vi "4310 DMM Measure.vi"(0 "IVI Refnum in":refnum<k15>, 1 "task in":refnum<k21>, 2 "Number of Samples in":i32, 3 "error in":errorcluster, 4 "gRPCid":T1) -> (7 "IVI Refnum out":refnum<k15>, 8 "task out":refnum<k21>, 9 "STOPSTREAM?":bool=TRUE, 10 "error out":errorcluster)   [LabVIEW 2019]
uses:
  VIs/grpcId.ctl
  QueryServer_AnalogInputData.ctl
  Global Operations.ctl
  <vilib>/DAQmx/read.llb/DAQmx Read (Analog 1D Wfm NChan NSamp).vi
  <vilib>/DAQmx/miscellaneous.llb/DAQmx Fill In Error Info.vi
  labview-grpc-query-server.lvlib
  <vilib>/NI_Real-Time Target Support.lvlib
  VIs/gprc-support.lvlib
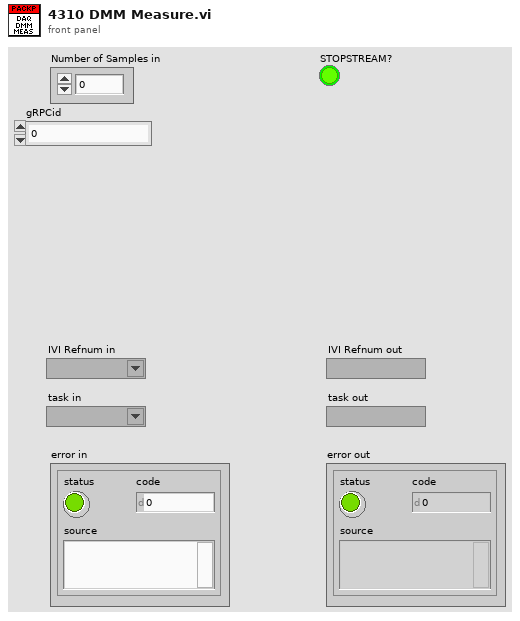
[diagram p1: front panel]
types:
  T1 = typedef "gprc-support.lvlib/grpcId.ctl" = u64
  T2 = typedef "Global Operations.ctl" = enum16{"Get", "Set"}
  T3 = typedef "labview-grpc-query-server.lvlib/QueryServer_AnalogInputData.ctl" = cluster{"RepeatedDMMValue":sgl[], "RepeatedDAQValue0":sgl[], "RepeatedDAQValue1":sgl[], "RepeatedDAQValue2":sgl[], "RepeatedDAQValue3":sgl[], "RepeatedDAQValue4":sgl[], "RepeatedDAQValue5":sgl[], "RepeatedDAQValue6":sgl[], "RepeatedDAQValue7":sgl[], "t0":string, "dt":sgl, "errorstatus":bool, "errorcode":i32, "errorsource":string}
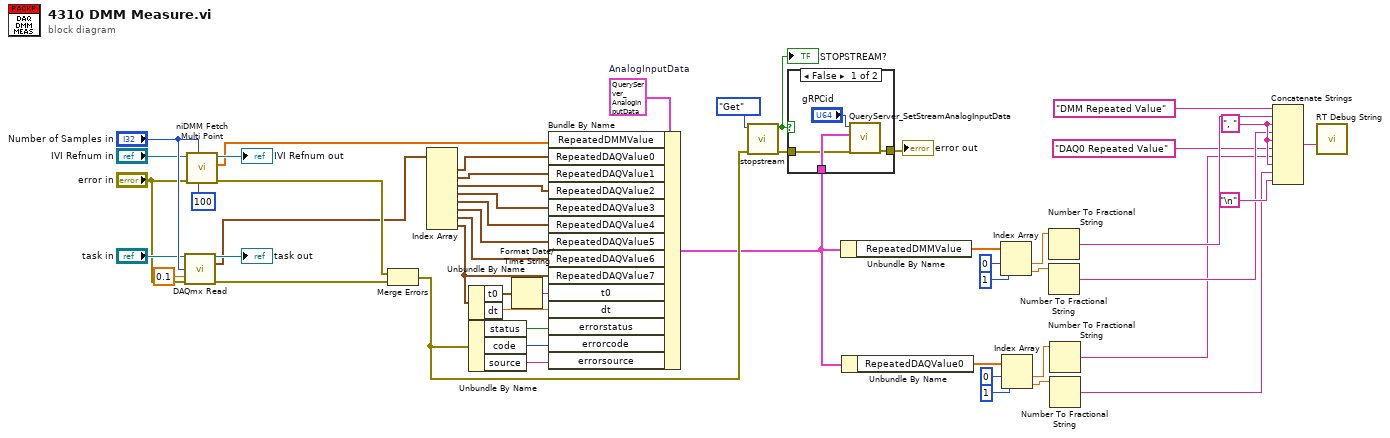
[diagram p0: block diagram]
diagram:
  w13 = ", "
  w43 = T3 {"RepeatedDMMValue"=[], "RepeatedDAQValue0"=[], "RepeatedDAQValue1"=[], "RepeatedDAQValue2"=[], "RepeatedDAQValue3"=[], "RepeatedDAQValue4"=[], "RepeatedDAQValue5"=[], "RepeatedDAQValue6"=[], "RepeatedDAQValue7"=[], "t0"="", "dt"=0.0, "errorstatus"=FALSE, "errorcode"=0, "errorsource"=""}  # AnalogInputData
  n1 = call-poly <vilib>:"DAQmx Read.vi"("task/channels in"="task in", "number of samples per channel"="Number of Samples in", "timeout"=0.1, "error in"="error in") -> ("task out"=→"task out":refnum<k21>, "data"=w29:waveform(dbl)[], "error out"=w45:errorcluster)  [unwired: 9 in]
  n2 = call <instrlib>:"niDMM Fetch Multi Point.vi"("Maximum Time (msec)"=100, "Number to Fetch"="Number of Samples in", "error in (no error)"="error in", "instrument handle"="IVI Refnum in") -> ("error out"=w44:errorcluster, "Measurements"=w30:dbl[], "instrument handle out"=→"IVI Refnum out":refnum<k15>)  [unwired: 4 in, 1 out]
  n3 = Merge Errors(w44, w45) -> (w21:errorcluster)
  n4 = Index Array(array=w29) -> (element #1=w42:waveform(dbl), element #2=w41:waveform(dbl), element #3=w40:waveform(dbl), element #4=w39:waveform(dbl), element #5=w38:waveform(dbl), element #6=w37:waveform(dbl), element #7=w36:waveform(dbl), element #8=w35:waveform(dbl))  [unwired: 8 in]
  n5 = Unbundle By Name(w35) -> ("t0"=w34:timestamp, "dt"=w32:dbl)
  n6 = Unbundle By Name(w21) -> ("status"=w27:bool, "code"=w31:i32, "source"=w26:string)
  n7 = Format Date/Time String(seconds (now)=w34) -> (date/time string=w33:string)  [unwired: 2 in]
  n8 = Bundle By Name(cluster=w43, "RepeatedDMMValue"=w30, "RepeatedDAQValue0"=w42, "RepeatedDAQValue1"=w41, "RepeatedDAQValue2"=w40, "RepeatedDAQValue3"=w39, "RepeatedDAQValue4"=w38, "RepeatedDAQValue5"=w37, "RepeatedDAQValue6"=w36, "RepeatedDAQValue7"=w35, "t0"=w33, "dt"=w32, "errorstatus"=w27, "errorcode"=w31, "errorsource"=w26) -> (w8:T3)
  n9 = call "stopstream.vi"("error in (no error)"=w21, "Operation"=Global_Operations."Get") -> ("error out"=w22:errorcluster, "STOPSTREAM?"=w23:bool)  [unwired: 8 in]
  "STOPSTREAM?" <- w23
  n10 = case shown="False" w23 {
    tunnel: w8 -> [w56 _]
    tunnel: [w54 w57] -> w25
    tunnel: w22 -> [w53 w57]
    frame False {
      n11 = call "QueryServer_SetStreamAnalogInputData.vi"("error in (no error)"=w53, "AnalogInputData"=w56, "gRPCid"="gRPCid") -> ("error out"=w54:errorcluster)  [unwired: 5 in, 1 out]
    }
    frame True {
    }
  }
  "error out" <- w25
  n12 = Unbundle By Name(w8) -> ("RepeatedDMMValue"=w20:sgl[])
  n13 = Unbundle By Name(w8) -> ("RepeatedDAQValue0"=w3:sgl[])
  n14 = Index Array(array=w20, index #1=0 ("index"), index #2=1 ("index")) -> (element #1=w16:sgl, element #2=w17:sgl)
  n15 = Index Array(array=w3, index #1=0 ("index"), index #2=1 ("index")) -> (element #1=w4:sgl, element #2=w5:sgl)
  n16 = Number To Fractional String(number=w16) -> (F-format string=w11:string)  [unwired: 3 in]
  n17 = Number To Fractional String(number=w17) -> (F-format string=w10:string)  [unwired: 3 in]
  n18 = Number To Fractional String(number=w4) -> (F-format string=w2:string)  [unwired: 3 in]
  n19 = Number To Fractional String(number=w5) -> (F-format string=w1:string)  [unwired: 3 in]
  n20 = Concatenate Strings("DMM Repeated Value" ("String to write"), w11, w13, w10, w13, "DAQ0 Repeated Value" ("string"), w2, w13, w1, "\n") -> (w14:string)
  n21 = call <vilib>:"RT Debug String.vi"("String to write"=w14) -> ()  [unwired: 10 in, 1 out]
